vi "solar_visa VISA Close.vi"(7 "Simulate? (F)":bool, 8 "error in (no error)":errorcluster, 10 "Ignore Error? (T)":bool=TRUE, 11 "VISA Resource in":refnum<visa-resource-name>) -> (0 "error out":errorcluster, 3 "VISA Resource out":refnum<visa-resource-name>)   [LabVIEW 2018]
doc: "This closes a VISA session. If <b>Ignore Error?</b> is true the error is ignored."
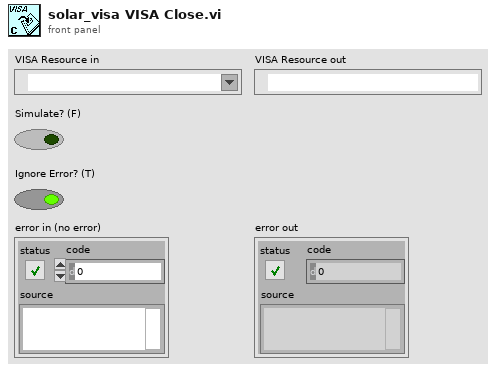
[diagram p1: front panel]
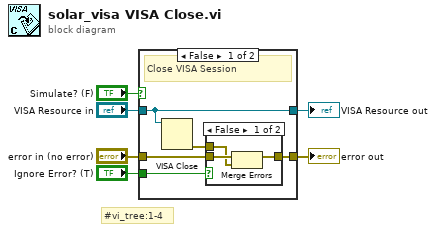
[diagram p0: block diagram]
diagram:
  # "#vi_tree:1-4"
  n1 = case shown="False" "Simulate? (F)" {
    tunnel: "error in (no error)" -> [w11 w16]
    tunnel: "VISA Resource in" -> [w10 w17]
    tunnel: [w9 w16] -> w4
    tunnel: [w10 w17] -> w3
    tunnel: "Ignore Error? (T)" -> [w7 _]
    frame False {
      # "Close VISA Session"
      n2 = VISA Close(VISA resource name=w10) -> (error out=w8:errorcluster)  [unwired: 1 in]
      n3 = case shown="False" w7 {
        tunnel: w11 -> [w14 w15]
        tunnel: [w13 w15] -> w9
        tunnel: w8 -> [w12 _]
        frame False {
          n4 = Merge Errors(w14, w12) -> (w13:errorcluster)
        }
        frame True {
        }
      }
    }
    frame True {
      # "Simulate - Do Nothing"
    }
  }
  "error out" <- w4
  "VISA Resource out" <- w3
